vi "Giroscópio_MPU6050-2.vi"() -> ()   [LabVIEW 2017]
uses:
  <vilib>/myRIO/Instrument Drivers/Onboard IO/I2C/typedefs/I2C User Configuration.ctl
  <vilib>/myRIO/Instrument Drivers/Onboard IO/I2C/typedefs/I2C Transfer Rate.ctl
  <vilib>/Platform/TimedLoop/XDataNode/timing_clust.ctl
  <vilib>/Platform/TimedLoop/XDataNode/nitl_modes.ctl
  <vilib>/Platform/TimedLoop/XDataNode/wakeup.ctl
  <vilib>/myRIO/Common/Instrument Driver Framework/myRIO v1.0/DIO/vis/myRIO v1.1 Open DIO.vi
  <vilib>/myRIO/Common/Instrument Driver Framework/myRIO v1.0/I2C/vis/myRIO v1.1 Open I2C.vi
  <vilib>/myRIO/Common/Instrument Driver Framework/myRIO v1.0/UART/vis/myRIO v1.0 Close UART.vi
  <vilib>/myRIO/Common/Instrument Driver Framework/Utilities/vis/Validate Channels.vi
  <vilib>/myRIO/Common/Instrument Driver Framework/myRIO v1.0/DIO/vis/myRIO v1.0 Reserve DIO.vi
  <vilib>/myRIO/Common/Instrument Driver Framework/myRIO v1.0/I2C/vis/myRIO v1.0 Reserve I2C.vi
  <vilib>/myRIO/Common/Instrument Driver Framework/myRIO v1.0/Resource Manager/vis/myRIO v1.0 Reserve Channel List.vi
  <vilib>/myRIO/Common/Instrument Driver Framework/myRIO v1.0/DIO/vis/myRIO v1.0 Build MUX Configuration DIO.vi
  <vilib>/myRIO/Common/Instrument Driver Framework/myRIO v1.0/I2C/vis/myRIO v1.0 Build MUX Configuration I2C.vi
  <vilib>/myRIO/Common/Instrument Driver Framework/myRIO v1.0/Resource Manager/vis/myRIO v1.0 Reserve Channel.vi
  <vilib>/myRIO/Common/Instrument Driver Framework/myRIO v1.0/Resource Manager/vis/myRIO v1.0 Unreserve Channel.vi
  <vilib>/myRIO/Common/Instrument Driver Framework/myRIO v1.0/Resource Manager/vis/myRIO v1.0 Create Configuration List.vi
  <vilib>/myRIO/Common/Instrument Driver Framework/myRIO v1.0/Resource Manager/vis/myRIO v1.0 Build Mutex Name.vi
  <vilib>/Utility/VariantDataType/GetNumericInfo.vi
  <vilib>/Utility/error.llb/Error Cluster From Error Code.vi
  <vilib>/myRIO/Common/Instrument Driver Framework/myRIO v1.0/myRIO v1.1 Open.vi
  <vilib>/myRIO/Common/Instrument Driver Framework/Utilities/vis/IO Manager.vi
  <vilib>/myRIO/Common/Instrument Driver Framework/Utilities/vis/Configuration Manager.vi
  <vilib>/myRIO/Common/Instrument Driver Framework/myRIO v1.0/Resource Manager/vis/myRIO v1.0 Configure IO.vi
  <vilib>/myRIO/Common/Instrument Driver Framework/myRIO v1.0/myRIO v1.0 Close.vi
  <vilib>/myRIO/Common/Instrument Driver Framework/myRIO v1.0/I2C/vis/myRIO v1.0 Configure I2C.vi
  <vilib>/myRIO/Common/Instrument Driver Framework/myRIO v1.0/I2C/vis/myRIO v1.0 Write I2C.vi
  <vilib>/myRIO/Common/Instrument Driver Framework/myRIO v1.0/DIO/vis/myRIO v1.0 Read DIO.vi
  <vilib>/myRIO/Common/Instrument Driver Framework/myRIO v1.0/I2C/vis/myRIO v1.0 Read I2C.vi
  <vilib>/myRIO/Common/Instrument Driver Framework/Utilities/vis/FPGA Ref Manager.vi
  <vilib>/myRIO/Common/Instrument Driver Framework/myRIO v1.0/myRIO v1.0 Reset FPGA.vi
  <vilib>/myRIO/Common/Instrument Driver Framework/myRIO v1.0/IRQ/vis/myRIO v1.0 IRQ Info FGV.vi
  <vilib>/myRIO/Common/Instrument Driver Framework/myRIO v1.0/IRQ/vis/myRIO v1.0 Timer IRQ Info FGV.vi
  <vilib>/myRIO/Common/Instrument Driver Framework/myRIO v1.0/IRQ/vis/myRIO v1.0 ISR Agent.vi
  <vilib>/Platform/TimedLoop/XDataNode/XDataNode.xnode
  <vilib>/myRIO/Instrument Drivers/Utilities/Utilities.lvlib
  <vilib>/myRIO/Instrument Drivers/Onboard IO/I2C/I2C.lvlib
  <vilib>/myRIO/Instrument Drivers/Onboard IO/DIO/DIO.lvlib
  <vilib>/Platform/TimedLoop/XDataNode/XDNodeRunTimeDep.lvlib
  <vilib>/ptbypt/NI_PtbyPt.lvlib
panel:
  out "Linear Acceleration [LSB/sec^2]":cluster{i16, i16, i16}(graph)
  out "Temp":i16
  out "Z acc":i16
  out "Y acc":i16
  out "X acc":i16
  in  "reset integrator":bool
  out "Z displacement":dbl format="%#_5g"
  out "Y displacement":dbl format="%#_5g"
  out "X displacement":dbl format="%#_5g"
  out "Angular displacement [LSB]":T1(graph)
  out "Angular rate [LSB/sec]":cluster{i16, i16, i16}(graph)
  out "Z rot rate":i16
  out "Y rot rate":i16
  out "X rot rate":i16
  in  "[ESC]":bool
  # "IMU demo"
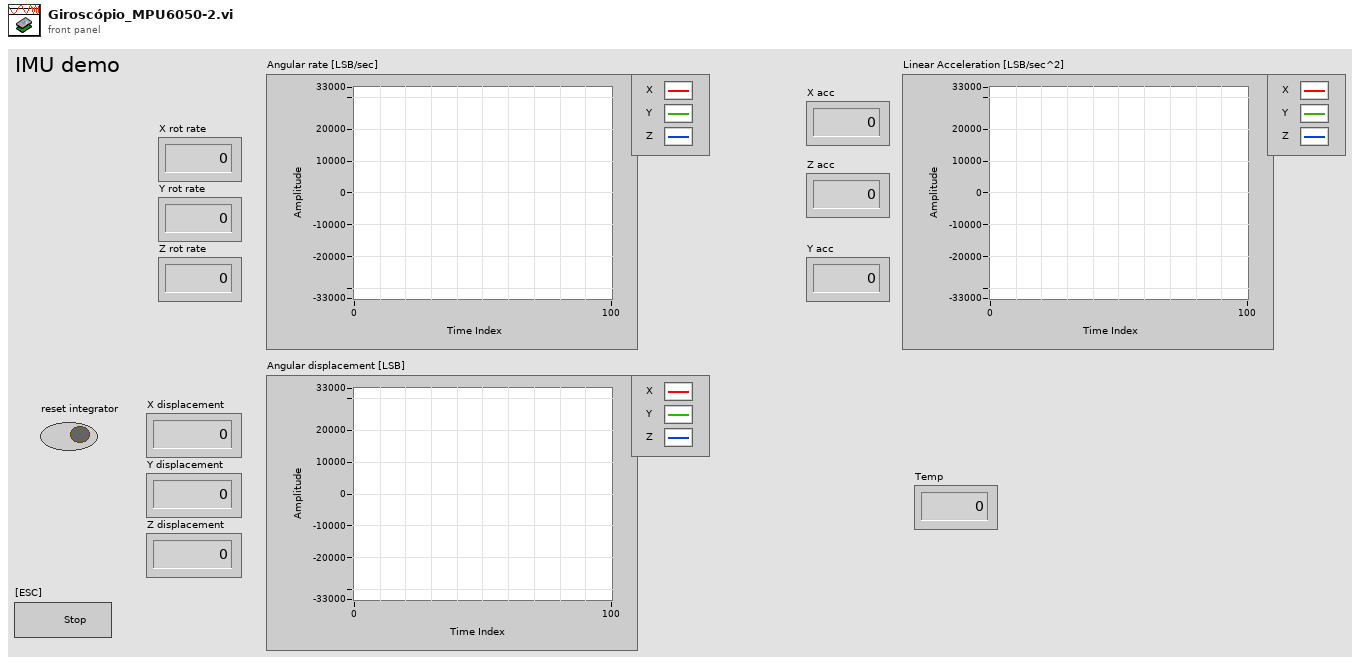
[diagram p1: front panel]
types:
  T1 = cluster{"integral x(t)":dbl, "integral x(t)":dbl, "integral x(t)":dbl}
  T2 = typedef "I2C.lvlib/I2C User Configuration.ctl" = cluster{"I2C Transfer Rate":T3}
  T3 = typedef "I2C.lvlib/I2C Transfer Rate.ctl" = enum16{"Standard mode (100 kbps)", "Fast mode (400 kbps)"}
  T4 = typedef "I2C.lvlib/I2C Reference.ctl" = cluster{"myRIO Reference":T5, "I2C Channels Enum":T9, "I2C Configuration":T10}
  T5 = typedef "myRIO Generic Hardware Reference.ctl" = cluster{"myRIO Model":T6, "myRIO Hardware Reference":T7}
  T6 = typedef "Hardware Version Enum.ctl" = enum16{"Unknown", "myRIO-1900", "myRIO-1950", "roboRIO", "NI ELVIS RIO CM"}
  T7 = typedef "myRIO v1.0 Reference.ctl" = cluster{"Generic FPGA Reference":T8, "Allow multiple opens":bool}
  T8 = typedef "Generic FPGA Reference.ctl" = refnum<k20>
  T9 = typedef "I2C Channels Enum.ctl" = enum16{"Not Connected", "A/I2C", "B/I2C", "I2C/I2C"}
  T10 = typedef "I2C.lvlib/I2C Configuration.ctl" = cluster{"I2C Transfer Rate":T3}
  T11 = typedef "DIO.lvlib/DIO Reference.ctl" = cluster{"myRIO Reference":T5, "DIO Channels List":T12}
  T12 = typedef "DIO Channels List.ctl" = T13[]
  T13 = typedef "DIO Channels Enum.ctl" = enum16{"Not Connected", "C/DIO0", "C/DIO1", "C/DIO2", "C/DIO3", "C/DIO4", "C/DIO5", "C/DIO6", "C/DIO7", "A/DIO0", "A/DIO1", "A/DIO2", "A/DIO3", "A/DIO4", "A/DIO5", "A/DIO6", "A/DIO7", "A/DIO8", "A/DIO9", "A/DIO10", "A/DIO11", "A/DIO12", "A/DIO13", "A/DIO14", "A/DIO15", "B/DIO0", "B/DIO1", "B/DIO2", "B/DIO3", "B/DIO4", "B/DIO5", "B/DIO6", "B/DIO7", "B/DIO8", "B/DIO9", "B/DIO10", "B/DIO11", "B/DIO12", "B/DIO13", "B/DIO14", "B/DIO15", "LED0", "LED1", "LED2", "LED3", "Button0", "DIO/DIO0", "DIO/DIO1", "DIO/DIO2", "DIO/DIO3", "DIO/DIO4", "DIO/DIO5", "DIO/DIO6", "DIO/DIO7", "DIO/DIO8", "DIO/DIO9", "SPI/CS0", "SPI/CS1", "SPI/CS2", "SPI/CS3", "LED RADIO (Green)", "LED RADIO (Red)", "LED COMM (Green)", "LED COMM (Red)", "LED MODE (Green)", "LED MODE (Red)"}
  T14 = typedef "XDNodeRunTimeDep.lvlib/timing_clust.ctl" = cluster{"Expected End [f-1]":u64, "Actual End [f-1]":u64, "Finished Late? [f-1]":bool, "Expected End [i-1]":u64, "Actual End [i-1]":u64, "Finished Late? [i-1]":bool, "Expected Start [i]":u64, "Actual Start [i]":u64, "Expected Start [f]":u64, "Actual Start [f]":u64, "Source Name":string, "Structure Name":string, "Period":i64, "Deadline":i64, "Offset":i64, "Start":i64, "Priority":i32, "Timeout":i32, "Mode":T15, "Wakeup Reason":T16, "Error":errorcluster, "Source Type":string, "Secondary Source Type":string, "Global End Time":u64, "Global Start Time":u64, "Frame Duration":u64, "Iteration Duration":u64, "Assigned CPU":i32, "I/O Scan Engine Mode":u32}
  T15 = typedef "XDNodeRunTimeDep.lvlib/nitl_modes.ctl" = enum32{"No Change", "Process missed periods, maintain original phase", "Discard missed periods, maintain original phase", "Process missed periods, ignore original phase", "Discard missed periods, ignore original phase"}
  T16 = typedef "XDNodeRunTimeDep.lvlib/wakeup.ctl" = enum32{"Normal", "Aborted", "Asynchronous wakeup", "Timing source error", "Timed loop error", "Timeout"}
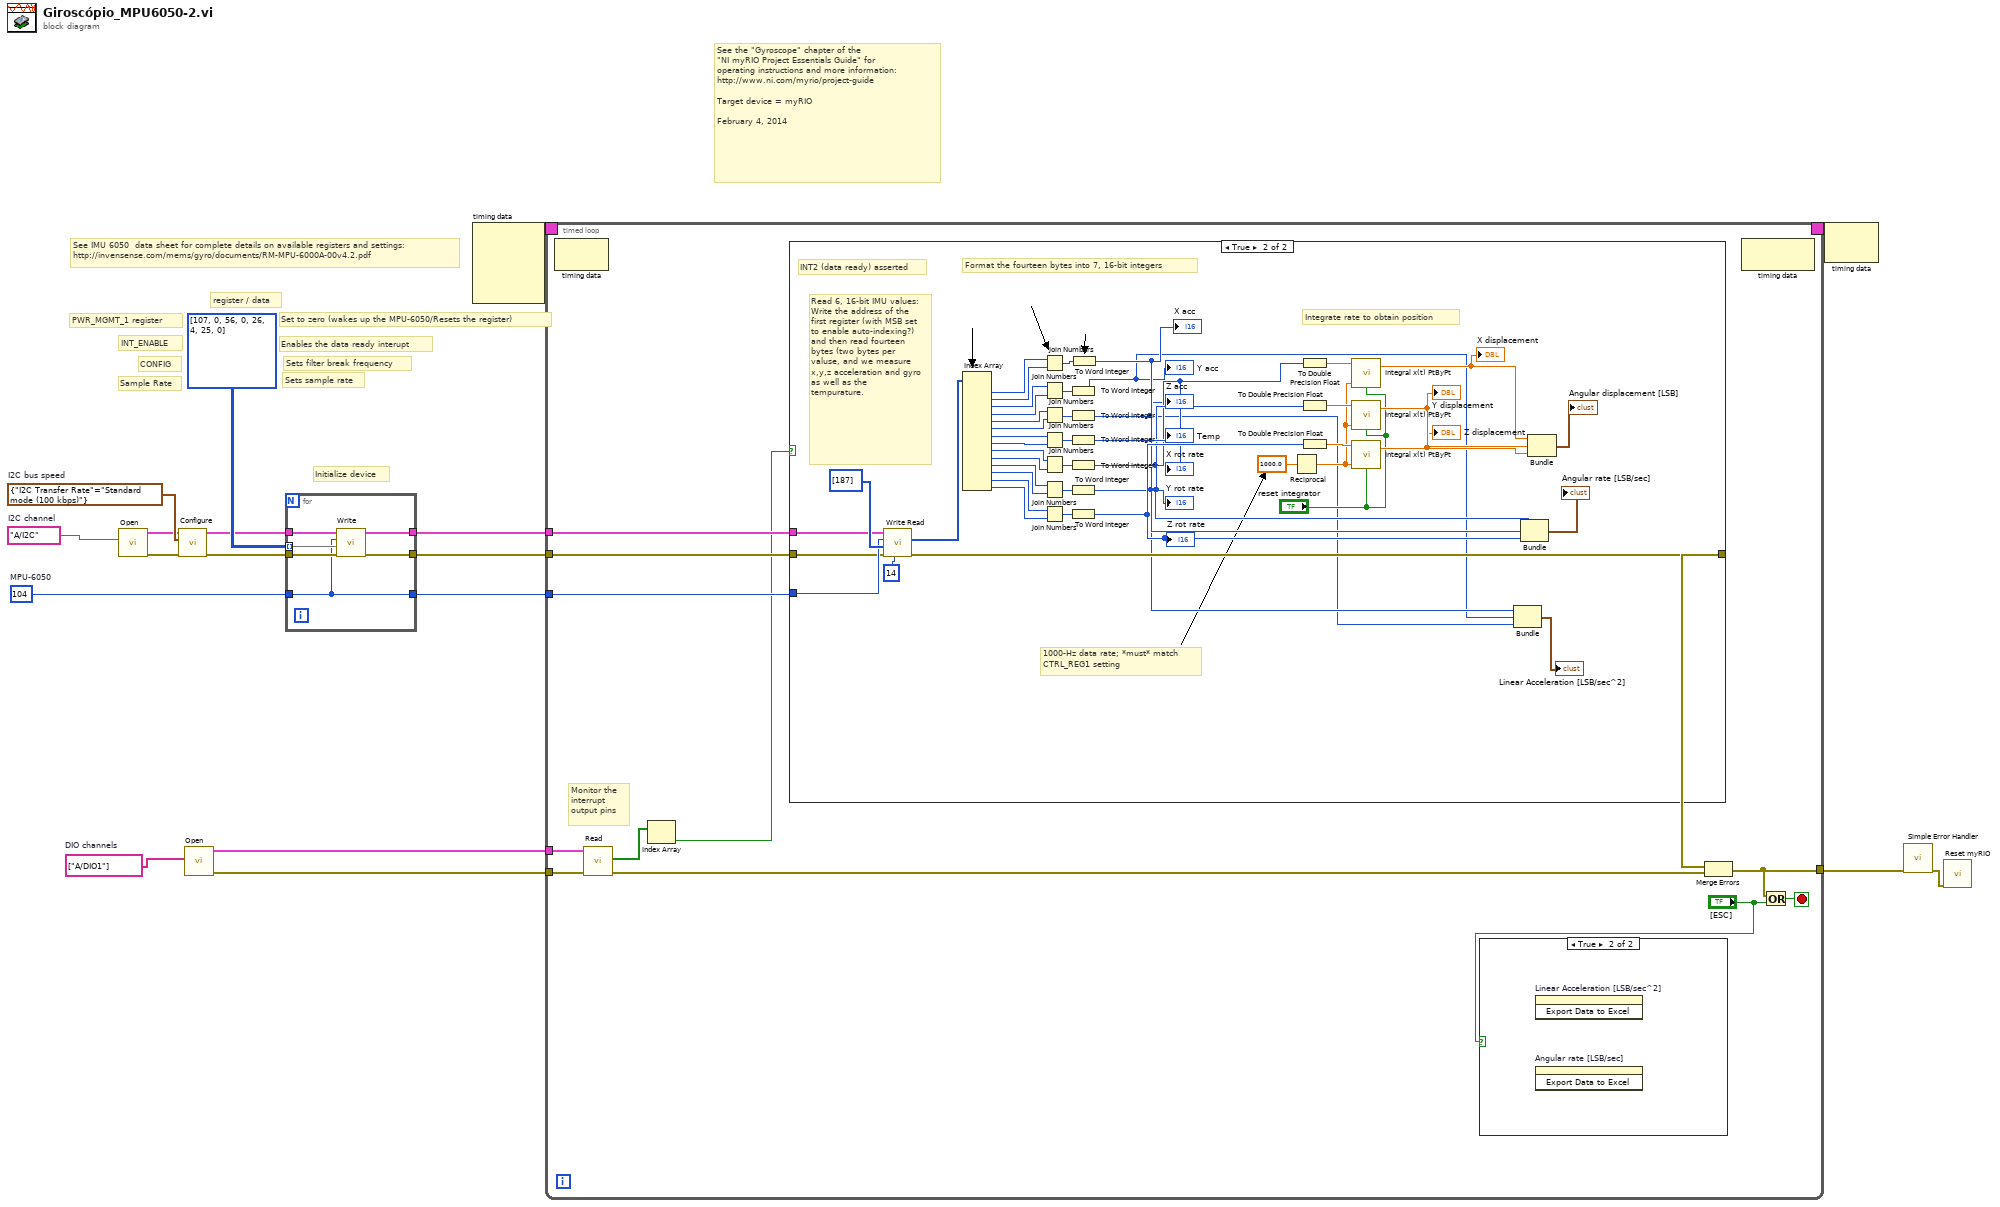
[diagram p0: block diagram]
diagram:
  w5 = tag[] ["A/DIO1"]  # DIO channels
  w16 = T2 {"I2C Transfer Rate"=enum."Standard mode (100 kbps)"}  # I2C bus speed
  w1 = tag "A/I2C"  # I2C channel
  w7 = u8 104  # MPU-6050
  # "Sets sample rate"
  # "Sample Rate"
  # "Sets filter break frequency"
  # "CONFIG"
  # "INT_ENABLE"
  # "Enables the data ready interupt"
  # "See the \"Gyroscope\" chapter of the\n\"NI myRIO Project Essentials Guide\" for\noperating instructions and more information: \nhttp://www.ni.com/myrio/project-guide\n\nTarget device = myRIO\n\nFebruary 4, 2014"
  # "Set to zero (wakes up the MPU-6050/Resets the register)"
  # "PWR_MGMT_1 register"
  # "Initialize device"
  # "See IMU 6050  data sheet for complete details on available registers and settings:\nhttp://invensense.com/mems/gyro/documents/RM-MPU-6000A-00v4.2.pdf"
  # "register / data"
  n1 = call <vilib>:"Open.vi"("Channel Name"=w1) -> ("error out"=w14:errorcluster, "I2C Ref Out"=w15:T4)  [unwired: 9 in]
  n2 = call <vilib>:"Configure.vi"("error in (no error)"=w14, "I2C User Configuration"=w16, "I2C Ref In"=w15) -> ("error out"=w8:errorcluster, "I2C Ref Out"=w9:T4)  [unwired: 7 in]
  n3 = call <vilib>:"Open.vi"("Channel Names"=w5) -> ("error out"=w6:errorcluster, "DIO Ref Out"=w2:T11)  [unwired: 9 in]
  n4 = for {
    tunnel: [w24] -> w13
    tunnel: [w23] -> w12
    tunnel: [w19] -> w11
    tunnel: u8[][] [[107, 0], [56, 0], [26, 4], [25, 0]] ("Bytes to Write") -> [w22] mode=indexing
    tunnel: w9 -> [w21]
    tunnel: w8 -> [w20]
    tunnel: w7 -> [w19]
    n5 = call <vilib>:"Write.vi"("error in (no error)"=w20, "Bytes to Write"=w22, "Slave Address (7-bit)"=w19, "I2C Ref In"=w21) -> ("error out"=w24:errorcluster, "I2C Ref Out"=w23:T4)  [unwired: 6 in]
  }
  n6 = node-c288() -> (w4:T14)  [unwired: 4 in]
  n7 = timed-loop {
    tunnel: [w28] -> w17
    tunnel: w11 -> [w33]
    tunnel: w13 -> [w35]
    tunnel: w12 -> [w34]
    tunnel: w6 -> [w32]
    timing: w4 -> [_]
    timing-out: [_] -> w3
    tunnel: w2 -> [w27]
    stop <- w36 stop-if-true
    # "Monitor the\ninterrupt\noutput pins"
    n8 = node-c288() -> ()  [unwired: 1 in, 1 out]
    n9 = call <vilib>:"Read.vi"("error in (no error)"=w32, "DIO Ref In"=w27) -> ("error out"=w26:errorcluster, "Values"=w29:bool[])  [unwired: 7 in, 1 out]
    n10 = Index Array "Index Array"(array=w29) -> (element=w30:bool)  [unwired: 1 in]
    n11 = case shown="True" w30 {
      tunnel: w35 -> [w39 w74]
      tunnel: w34 -> [_ w75]
      tunnel: w33 -> [_ w81]
      tunnel: [w39 w80] -> w31
      frame False {
        # "INT2 (data ready) deasserted"
      }
      frame True {
        # "1000-Hz data rate; *must* match\nCTRL_REG1 setting"
        # "Integrate rate to obtain position"
        # "INT2 (data ready) asserted"
        # "Read 6, 16-bit IMU values:\nWrite the address of the first register (with MSB set to enable auto-indexing?) and then read fourteen bytes (two bytes per valuse, and we measure x,y,z acceleration and gyro as well as the tempurature."
        # "Format the fourteen bytes into 7, 16-bit integers"
        n12 = call <vilib>:"Write Read.vi"("Byte Count"=u32 14, "error in (no error)"=w74, "Bytes to Write"=u8[] [187], "Slave Address (7-bit)"=w81, "I2C Ref In"=w75) -> ("error out"=w80:errorcluster, "Bytes Read"=w79:u8[])  [unwired: 3 in, 1 out]
        n13 = Index Array "Index Array"(array=w79) -> (element #1=w66:u8, element #2=w65:u8, element #3=w64:u8, element #4=w63:u8, element #5=w62:u8, element #6=w61:u8, element #7=w60:u8, element #8=w59:u8, element #9=w58:u8, element #10=w57:u8, element #11=w56:u8, element #12=w55:u8, element #13=w54:u8, element #14=w53:u8)  [unwired: 14 in]
        n14 = Join Numbers(hi=w66, lo=w65) -> ((hi.lo)=w86:u16)
        n15 = Join Numbers(hi=w64, lo=w63) -> ((hi.lo)=w85:u16)
        n16 = Join Numbers(hi=w62, lo=w61) -> ((hi.lo)=w84:u16)
        n17 = Join Numbers(hi=w60, lo=w59) -> ((hi.lo)=w52:u16)
        n18 = Join Numbers(hi=w58, lo=w57) -> ((hi.lo)=w51:u16)
        n19 = Join Numbers(hi=w56, lo=w55) -> ((hi.lo)=w50:u16)
        n20 = Join Numbers(hi=w54, lo=w53) -> ((hi.lo)=w49:u16)
        n21 = To Word Integer(number=w85) -> (16bit integer=w41:i16)
        "Y acc" <- w41
        n22 = To Word Integer(number=w84) -> (16bit integer=w40:i16)
        "Z acc" <- w40
        n23 = To Word Integer(number=w52) -> (16bit integer=→"Temp":i16)
        n24 = To Word Integer(number=w51) -> (16bit integer=w44:i16)
        "X rot rate" <- w44
        n25 = To Word Integer(number=w50) -> (16bit integer=w45:i16)
        "Y rot rate" <- w45
        n26 = To Word Integer(number=w49) -> (16bit integer=w46:i16)
        "Z rot rate" <- w46
        n27 = To Word Integer(number=w86) -> (16bit integer=w42:i16)
        "X acc" <- w42
        n28 = Reciprocal(x=1000.0 ("dt")) -> (1/x=w72:dbl)
        n29 = To Double Precision Float(number=w44) -> (double precision float=w67:dbl)
        n30 = To Double Precision Float(number=w45) -> (double precision float=w78:dbl)
        n31 = To Double Precision Float(number=w46) -> (double precision float=w77:dbl)
        n32 = call <vilib>:"Integral x(t) PtByPt.vi"("initialize"="reset integrator", "dt"=w72, "x"=w67) -> ("integral x(t)"=w68:dbl)  [unwired: 1 in, 1 out]
        "X displacement" <- w68
        n33 = call <vilib>:"Integral x(t) PtByPt.vi"("initialize"="reset integrator", "dt"=w72, "x"=w78) -> ("integral x(t)"=w71:dbl)  [unwired: 1 in, 1 out]
        "Y displacement" <- w71
        n34 = call <vilib>:"Integral x(t) PtByPt.vi"("initialize"="reset integrator", "dt"=w72, "x"=w77) -> ("integral x(t)"=w70:dbl)  [unwired: 1 in, 1 out]
        "Z displacement" <- w70
        n35 = Bundle "Bundle"(w42, w41, w40) -> (→"Linear Acceleration [LSB/sec^2]":cluster{i16, i16, i16})  [unwired: 1 in]
        n36 = Bundle "Bundle"(w44, w45, w46) -> (→"Angular rate [LSB/sec]":cluster{i16, i16, i16})  [unwired: 1 in]
        n37 = Bundle "Bundle"("integral x(t)"=w68, "integral x(t)"=w71, "integral x(t)"=w70) -> (→"Angular displacement [LSB]":T1)  [unwired: 1 in]
      }
    }
    n38 = case shown="True" "[ESC]" {
      frame False {
      }
      frame True {
        n39 = invoke on="Linear Acceleration [LSB/sec^2]" class="WFChart (strict)" method="Export Data to Excel"() -> ()  [unwired: 3 in, 3 out]
        n40 = invoke on="Angular rate [LSB/sec]" class="WFChart (strict)" method="Export Data to Excel"() -> ()  [unwired: 3 in, 3 out]
      }
    }
    n41 = Merge Errors "Merge Errors"(w31, w26) -> (w28:errorcluster)
    n42 = node-c288() -> ()  [unwired: 1 in, 1 out]
    n43 = Or(x=w28, y="[ESC]") -> (x .or. y?=w36:bool)
  }
  n44 = node-c288(w3) -> ()  [unwired: 1 out]
  n45 = call <vilib>:"Simple Error Handler.vi"("error in (no error)"=w17) -> ("error out"=w18:errorcluster)  [unwired: 4 in, 4 out]
  n46 = call <vilib>:"Reset myRIO.vi"("error in (no error)"=w18) -> ()  [unwired: 10 in, 1 out]
